vi "CheckSettings.vi"(0 "ChromaAcLoad in":refnum<class "ChromaAcLoad.lvclass">, 1 "RangeCheck":T1, 2 "Phase":i32, 3 "error in (no error)":errorcluster) -> (7 "ChromaAcLoad out":refnum<class "ChromaAcLoad.lvclass">, 10 "error out":errorcluster)   [LabVIEW 2018, in "AcPwrPlugins.lvlib" / "ChromaAcLoad.lvclass"]
doc: "This VI checks the value of the instrument settings and returns an error if the value is outside the instrument range."
uses:
  ChromaAcLoad.lvclass
  C:/Users/ico/Documents/Projects/NistPluggableModules/AcPwr/AcPwrPlugins/AcPwrBaseClass/AcPwrBase.lvclass
  TypeDefs/RangeCheck.ctl
  AcPwrBaseClass/AcPwrBase.lvclass/AcPwrBase.ctl
  AcPwrBaseClass/Accessors/Read BaseConfig.vi
  <vilib>/Utility/error.llb/Error Cluster From Error Code.vi
  <vilib>/ErrorRing/Error Ring.xnode
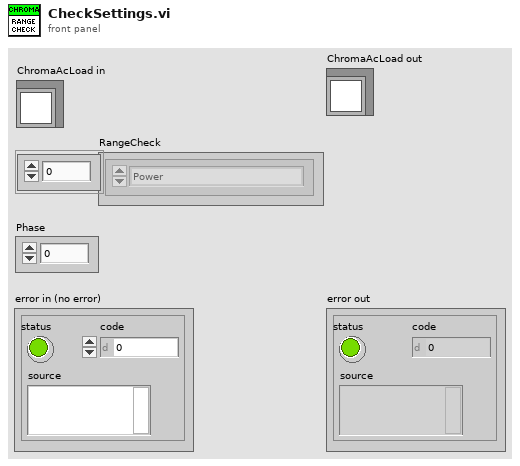
[diagram p1: front panel]
types:
  T1 = typedef "AcPwrPlugins.lvlib/ChromaAcLoad.lvclass/RangeCheck.ctl" = enum16{"Power", "Power Limit", "Current", "Current Peak", "Current Limit", "Voltage", "AC Resistance", "DC Resistance", "Frequency", "Crest Factor", "Power Factor", "RLC Power Factor", "Rise Slew Rate", "Fall Slew Rate", "Capacitance", "Inductance", "Parallel Resistance", "Series Resistance"}[]
  T2 = typedef "AcPwrPlugins.lvlib/AcPwrBase.lvclass/BaseConfig.ctl" = cluster{"Frequency":dbl, "FrequencyRange":dbl[], "Phases":T3[], "Name":string, "Chroma":T4, "NHRDC":T5, "PPS":T6, "PluginConfigVariant":variant}
  T3 = typedef "AcPwrPlugins.lvlib/AcPwrBase.lvclass/Phase.ctl" = cluster{"Name":string, "Enabled":bool, "VoltageLevel":dbl, "Handle":string, "VoltageRange":dbl[], "Connected":bool, "CurrentLimit":dbl, "Waveform":string}
  T4 = typedef "AcPwrPlugins.lvlib/ChromaAcLoad.lvclass/DeviceProperties.ctl" = cluster{"Configuration Mode":enum16{"Constant Voltage (DC)", "Constant Power (DC)", "Constant Power (AC)", "Constant Current (DC)", "Constant Current (AC)", "Constant Resistance (DC)", "Constant Resistance (AC)", "Rectified Mode (DC)", "Inrush (AC)", "RLC CP (AC)", "RLC (AC)"}, "Phases":cluster{"Handle":string, "Name":string, "Phase Select":i32, "Instrument Options":string, "id query (T)":bool, "reset device (T)":bool, "Load Short Circuited":bool, "Line Synchronization":bool, "Load Current (A/Arms)":dbl, "Load Voltage (V/Vrms)":dbl, "Load Power (W)":dbl, "Load Resistance (Ohms)":dbl, "Load Current Peak Limit (A)":dbl, "Load Current Limit (A/Arms)":dbl, "Load Power Limit (W)":dbl, "Synch Frequency (Hz)":dbl, "Priority":enum16{"CF Only", "PF Only", "Both (CF)", "Both (PF)"}, "Crest Factor":dbl, "Power Factor":dbl, "Slew Rate":cluster{"Rise Slew Rate (A/ms)":i32, "Fall Slew Rate (A/ms)":i32}, "LC/RLC Mode":cluster{"Capacitance (uF)":i32, "Inductance (uH)":i32, "Series Resistance (Ohm)":dbl, "Parallel Resistance (Ohm)":dbl}, "Timing":cluster{"TimingOn":enum16{""}, "Hours":u32, "Minutes":u32, "Seconds":dbl, "CutoffVoltage":dbl}, "Connected":bool}[]}
  T5 = typedef "AcPwrPlugins.lvlib/NHRDCPower.lvclass/Device(s)Settings.ctl" = cluster{"Handle":string, "Name":string, "id query (Yes)":bool, "reset device (Yes)":bool, "Connected":bool, "Initial Battery Detect Voltage (0)":sgl, "SafetySettings":cluster{"SetWatchDog":bool, "Voltage (V)":sgl, "Current (A)":sgl, "Power (W)":sgl, "Voltage Delay (s)":sgl, "Current Delay (s)":sgl, "Power Delay (s)":sgl}, "Options String":string, "Aperture Time (s)":sgl, "operating state (Off)":i32, "OutputSettings":cluster{"Voltage (V)":sgl, "Current (A)":sgl, "Resistance (Ohms)":sgl, "Power (W)":sgl, "Enable Voltage":bool, "Enable Current":bool, "Enable Resistance":bool, "Enable Power":bool, "Delay After (s)":sgl, "Wait Value (V, A, W)":sgl, "Enable Wait":bool, "Wait on Value":i32}[], "SlewRate":cluster{"Set Voltage Rate V/S":dbl, "Set Current Rate A/S":dbl, "Set Resistance Rate R/S":dbl, "Set Power Rate W/S":dbl}}[]
  T6 = typedef "AcPwrPlugins.lvlib/PacificPowerSource.lvclass/DeviceSettings.ctl" = cluster{"Handle":string, "Connected":bool, "Clear Device (F)":bool, "btnIdQuery":bool, "btnReset":bool, "Program #":cluster{"Phase B (Degrees)":i32, "Waveform A (1: Sine)":i32, "Voltage Level (Va)":dbl, "Program Number (0)":i32, "Voltage Level (Vb) ":dbl, "Form (3: Three)":u16, "Coupling  (0: Direct)":u16, "Frequency (45Hz)":dbl, "Current Limit (40A)":dbl, "Phase C (Degrees)":i32, "Voltage Level (Vc)":dbl, "Waveform B (1: Sine)":i32, "Waveform C (1: Sine)":i32}[], "Impedance Parameters (off, 0.00)":cluster{"State":bool, "Impedance":dbl}, "Transient Execution (F)":bool, "OutputEnabled":bool, "Source Range":cluster{"Frequency Minimum (45 Hz)":dbl, "Frequency Maximum (1200 Hz)":dbl, "Voltage Maximum (V)":dbl, "Voltage Minimum (V)":dbl, "Range Control (0: Auto)":u16, "Initial Voltage (0V)":u16, "Frequency Range (600Hz)":u16}, "Port Type":enum16{"GPIB", "Serial"}}[]
  T7 = cluster{"Handle":string, "Name":string, "Phase Select":i32, "Instrument Options":string, "id query (T)":bool, "reset device (T)":bool, "Load Short Circuited":bool, "Line Synchronization":bool, "Load Current (A/Arms)":dbl, "Load Voltage (V/Vrms)":dbl, "Load Power (W)":dbl, "Load Resistance (Ohms)":dbl, "Load Current Peak Limit (A)":dbl, "Load Current Limit (A/Arms)":dbl, "Load Power Limit (W)":dbl, "Synch Frequency (Hz)":dbl, "Priority":enum16{"CF Only", "PF Only", "Both (CF)", "Both (PF)"}, "Crest Factor":dbl, "Power Factor":dbl, "Slew Rate":cluster{"Rise Slew Rate (A/ms)":i32, "Fall Slew Rate (A/ms)":i32}, "LC/RLC Mode":cluster{"Capacitance (uF)":i32, "Inductance (uH)":i32, "Series Resistance (Ohm)":dbl, "Parallel Resistance (Ohm)":dbl}, "Timing":cluster{"TimingOn":enum16{""}, "Hours":u32, "Minutes":u32, "Seconds":dbl, "CutoffVoltage":dbl}, "Connected":bool}[]
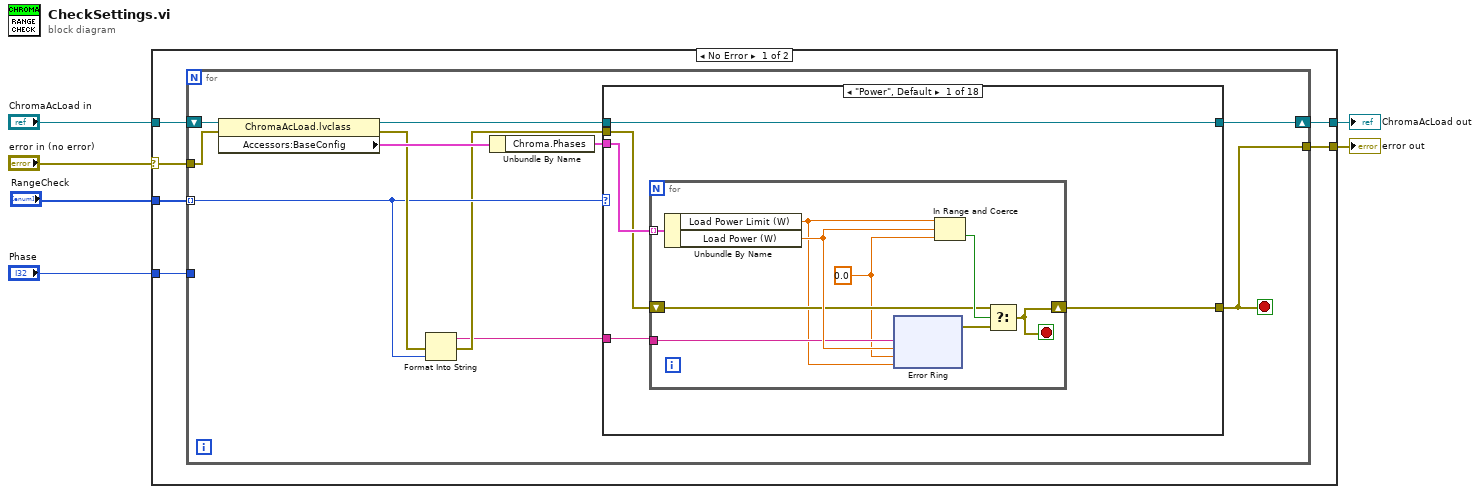
[diagram p0: block diagram]
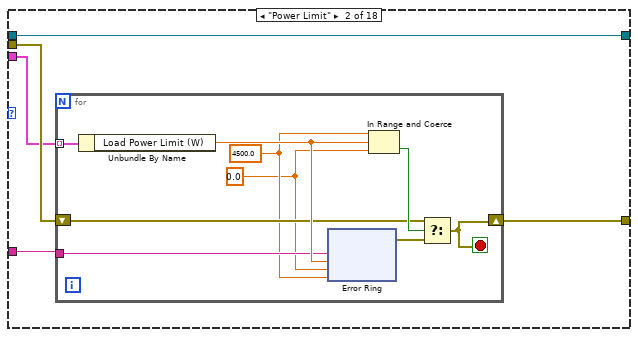
[diagram p2: hidden frame]
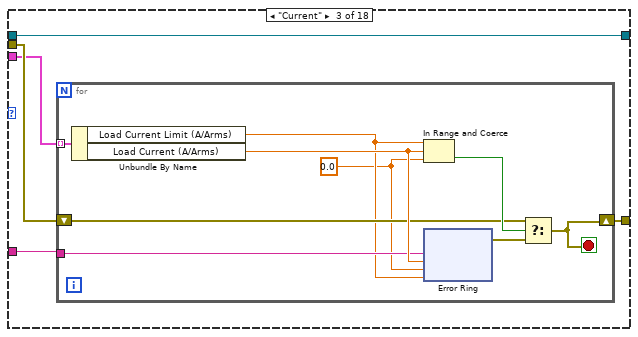
[diagram p3: hidden frame]
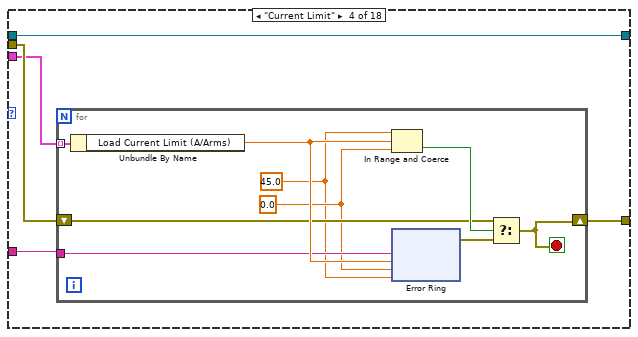
[diagram p4: hidden frame]
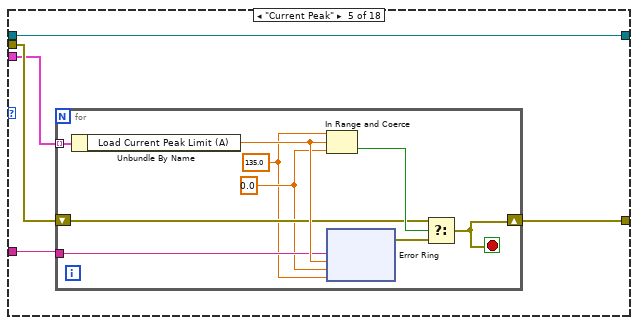
[diagram p5: hidden frame]
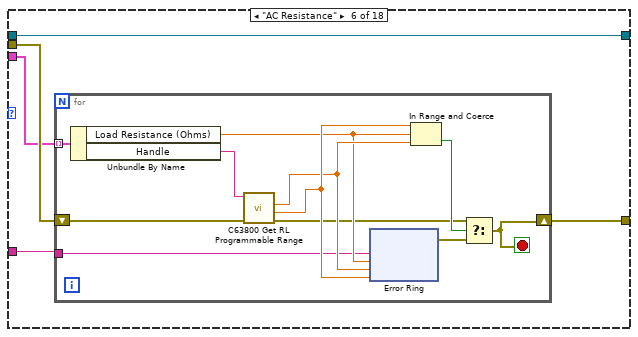
[diagram p6: hidden frame]
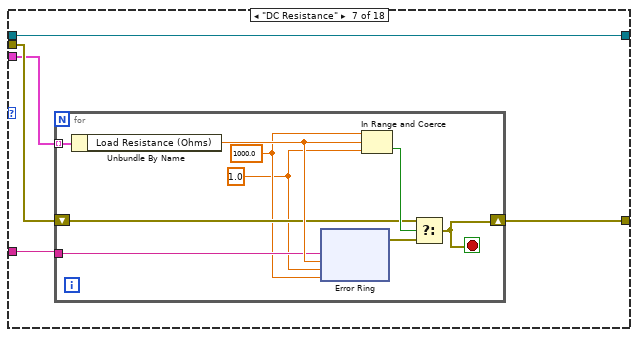
[diagram p7: hidden frame]
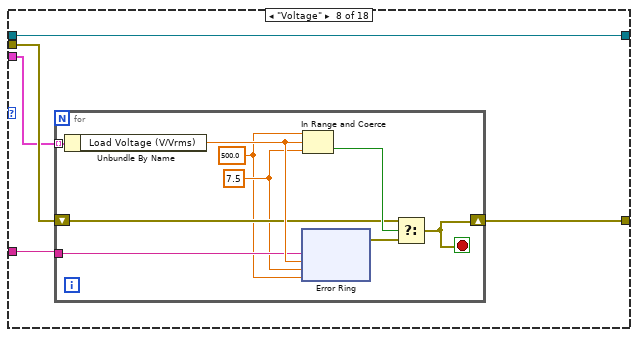
[diagram p8: hidden frame]
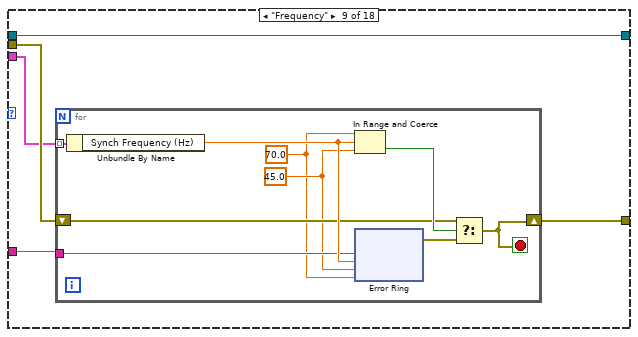
[diagram p9: hidden frame]
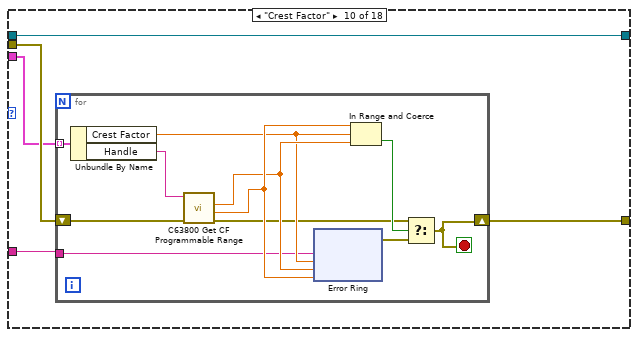
[diagram p10: hidden frame]
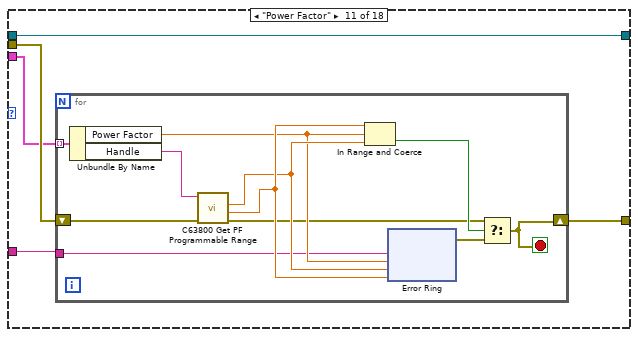
[diagram p11: hidden frame]
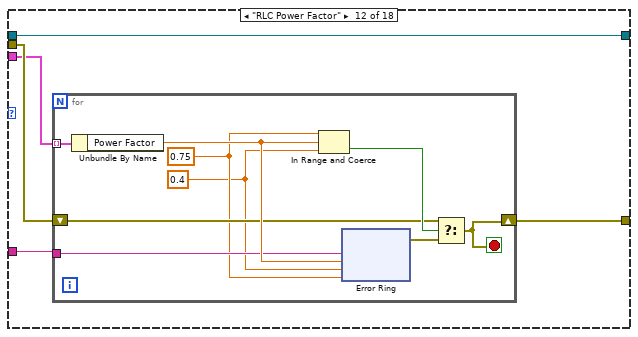
[diagram p12: hidden frame]
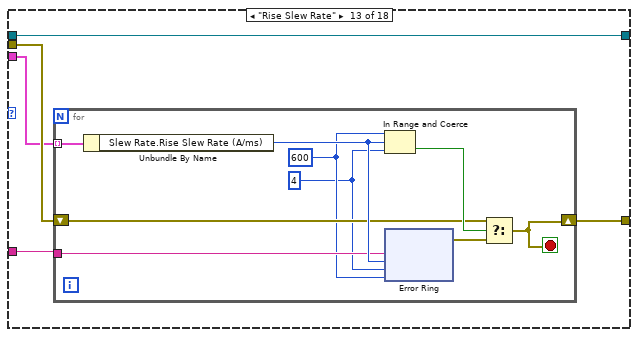
[diagram p13: hidden frame]
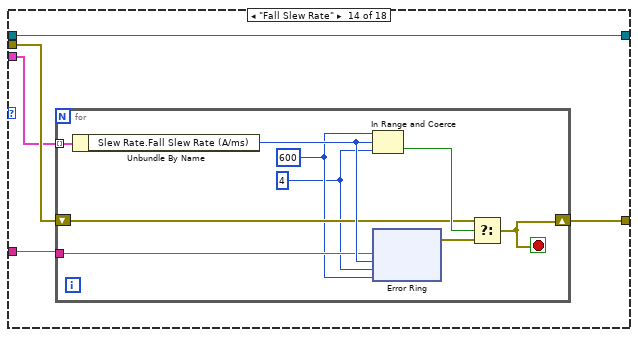
[diagram p14: hidden frame]
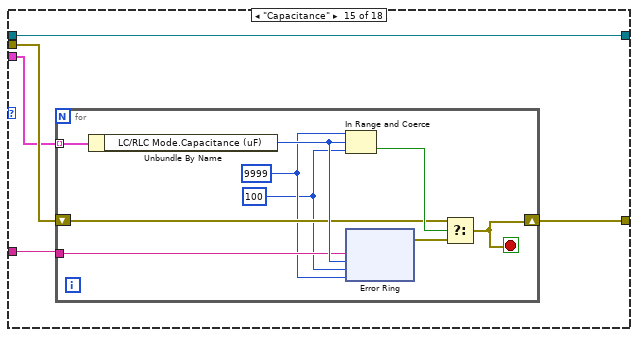
[diagram p15: hidden frame]
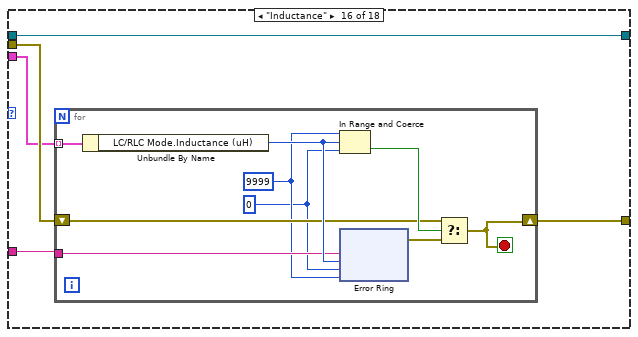
[diagram p16: hidden frame]
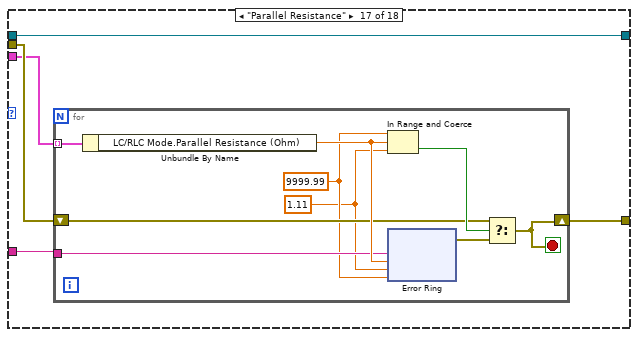
[diagram p17: hidden frame]
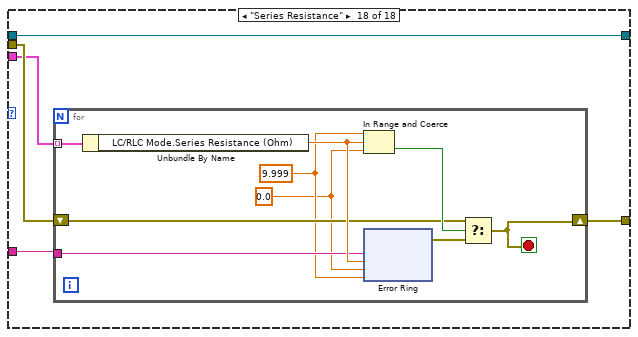
[diagram p18: hidden frame]
diagram:
  n1 = case shown="No Error" "error in (no error)" {
    selector: "error in (no error)" -> [w9 w462]
    tunnel: "ChromaAcLoad in" -> [w12 w463]
    tunnel: "Phase" -> [w11 _]
    tunnel: [w10 w463] -> w4
    tunnel: "RangeCheck" -> [w8 _]
    tunnel: [w7 w462] -> w1
    frame No Error {
      n2 = for {
        tunnel: w11 -> [_]
        shift-right: [w22] -> w10
        shift-left: w12 -> [w20]
        tunnel: w9 -> [w23]
        tunnel: w8 -> [w15] mode=indexing
        tunnel: [w21] -> w7
        stop <- w21 stop-if-true
        n3 = property class="ChromaAcLoad.lvclass"(reference=w20, error in=w23) -> (reference out=w19:refnum<class "ChromaAcLoad.lvclass">, error out=w16:errorcluster, "Accessors:BaseConfig"=w18:T2)
        n4 = Format Into String(error in=w16, w15) -> (resulting string=w13:string, error out=w14:errorcluster)  [unwired: 2 in]
        n5 = Unbundle By Name(w18) -> ("Chroma.Phases"=w17:T7)
        n6 = case shown="\"Power\", Default" w15 {
          tunnel: w19 -> [w28 w52 w76 w100 w124 w148 w174 w198 w222 w246 w272 w298 w322 w346 w370 w394 w418 w442]
          tunnel: w14 -> [w24 w51 w75 w99 w123 w147 w173 w197 w221 w245 w271 w297 w321 w345 w369 w393 w417 w441]
          tunnel: [w28 w52 w76 w100 w124 w148 w174 w198 w222 w246 w272 w298 w322 w346 w370 w394 w418 w442] -> w22
          tunnel: [w27 w50 w74 w98 w122 w146 w172 w196 w220 w244 w270 w296 w320 w344 w368 w392 w416 w440] -> w21
          tunnel: w17 -> [w26 w49 w73 w96 w121 w145 w170 w194 w218 w242 w268 w294 w319 w343 w366 w391 w414 w438]
          tunnel: w13 -> [w25 w48 w72 w97 w120 w144 w171 w195 w219 w243 w269 w295 w318 w342 w367 w390 w415 w439]
          frame "Power", Default {
            n7 = for {
              shift-right: [w34] -> w27
              shift-left: w24 -> [w32]
              tunnel: w26 -> [w36] mode=indexing
              tunnel: w25 -> [w31]
              stop <- w34 stop-if-true
              w29 = 0.0 ("Load Power Limit (W)")
              n8 = Unbundle By Name(w36) -> ("Load Power Limit (W)"=w30:dbl, "Load Power (W)"=w33:dbl)
              n9 = xnode "Error Ring"("parameter 0"=w31, "parameter 1"=w33, "parameter 2"=w29, "parameter 3"=w30) -> ("error out"=w37:errorcluster)
              n10 = In Range and Coerce(upper limit=w30, x=w33, lower limit=w29) -> (In Range?=w35:bool)  [unwired: 1 out]
              n11 = Select(t=w32, s=w35, f=w37) -> (s? t:f=w34:errorcluster)
            }
          }
          frame "Power Limit" {
            n12 = for {
              shift-right: [w58] -> w50
              shift-left: w51 -> [w56]
              tunnel: w49 -> [w60] mode=indexing
              tunnel: w48 -> [w55]
              stop <- w58 stop-if-true
              w54 = 4500.0
              w53 = 0.0
              n13 = Unbundle By Name(w60) -> ("Load Power Limit (W)"=w57:dbl)
              n14 = xnode "Error Ring"("parameter 0"=w55, "parameter 1"=w57, "parameter 2"=w53, "parameter 3"=w54) -> ("error out"=w61:errorcluster)
              n15 = In Range and Coerce(upper limit=w54, x=w57, lower limit=w53) -> (In Range?=w59:bool)  [unwired: 1 out]
              n16 = Select(t=w56, s=w59, f=w61) -> (s? t:f=w58:errorcluster)
            }
          }
          frame "Current" {
            n17 = for {
              shift-right: [w82] -> w74
              shift-left: w75 -> [w80]
              tunnel: w73 -> [w84] mode=indexing
              tunnel: w72 -> [w79]
              stop <- w82 stop-if-true
              w77 = 0.0 ("Load Current (A/Arms)")
              n18 = Unbundle By Name(w84) -> ("Load Current Limit (A/Arms)"=w78:dbl, "Load Current (A/Arms)"=w81:dbl)
              n19 = In Range and Coerce(upper limit=w78, x=w81, lower limit=w77) -> (In Range?=w83:bool)  [unwired: 1 out]
              n20 = xnode "Error Ring"("parameter 0"=w79, "parameter 1"=w81, "parameter 2"=w77, "parameter 3"=w78) -> ("error out"=w85:errorcluster)
              n21 = Select(t=w80, s=w83, f=w85) -> (s? t:f=w82:errorcluster)
            }
          }
          frame "Current Limit" {
            n22 = for {
              shift-right: [w106] -> w98
              shift-left: w99 -> [w104]
              tunnel: w96 -> [w108] mode=indexing
              tunnel: w97 -> [w103]
              stop <- w106 stop-if-true
              w101 = 45.0
              w102 = 0.0
              n23 = Unbundle By Name(w108) -> ("Load Current Limit (A/Arms)"=w105:dbl)
              n24 = In Range and Coerce(upper limit=w101, x=w105, lower limit=w102) -> (In Range?=w107:bool)  [unwired: 1 out]
              n25 = xnode "Error Ring"("parameter 0"=w103, "parameter 1"=w105, "parameter 2"=w102, "parameter 3"=w101) -> ("error out"=w109:errorcluster)
              n26 = Select(t=w104, s=w107, f=w109) -> (s? t:f=w106:errorcluster)
            }
          }
          frame "Current Peak" {
            n27 = for {
              shift-right: [w130] -> w122
              shift-left: w123 -> [w128]
              tunnel: w121 -> [w132] mode=indexing
              tunnel: w120 -> [w127]
              stop <- w130 stop-if-true
              w125 = 135.0
              w126 = 0.0
              n28 = Unbundle By Name(w132) -> ("Load Current Peak Limit (A)"=w129:dbl)
              n29 = In Range and Coerce(upper limit=w125, x=w129, lower limit=w126) -> (In Range?=w131:bool)  [unwired: 1 out]
              n30 = xnode "Error Ring"("parameter 0"=w127, "parameter 1"=w129, "parameter 2"=w126, "parameter 3"=w125) -> ("error out"=w133:errorcluster)
              n31 = Select(t=w128, s=w131, f=w133) -> (s? t:f=w130:errorcluster)
            }
          }
          frame "AC Resistance" {
            n32 = for {
              shift-right: [w154] -> w146
              shift-left: w147 -> [w152]
              tunnel: w145 -> [w158] mode=indexing
              tunnel: w144 -> [w149]
              stop <- w154 stop-if-true
              n33 = Unbundle By Name(w158) -> ("Load Resistance (Ohms)"=w153:dbl, "Handle"=w150:string)
              n34 = call <instrlib>:"C63800 Get RL Programmable Range.vi"("error in (no error)"=w152, "Instrument Handle"=w150) -> ("error out"=w151:errorcluster, "Maximum"=w157:dbl, "Minimum"=w156:dbl)  [unwired: 6 in, 1 out]
              n35 = xnode "Error Ring"("parameter 0"=w149, "parameter 1"=w153, "parameter 2"=w156, "parameter 3"=w157) -> ("error out"=w159:errorcluster)
              n36 = In Range and Coerce(upper limit=w157, x=w153, lower limit=w156) -> (In Range?=w155:bool)  [unwired: 1 out]
              n37 = Select(t=w151, s=w155, f=w159) -> (s? t:f=w154:errorcluster)
            }
          }
          frame "DC Resistance" {
            n38 = for {
              shift-right: [w180] -> w172
              shift-left: w173 -> [w178]
              tunnel: w170 -> [w182] mode=indexing
              tunnel: w171 -> [w177]
              stop <- w180 stop-if-true
              w176 = 1000.0
              w175 = 1.0
              n39 = Unbundle By Name(w182) -> ("Load Resistance (Ohms)"=w179:dbl)
              n40 = xnode "Error Ring"("parameter 0"=w177, "parameter 1"=w179, "parameter 2"=w175, "parameter 3"=w176) -> ("error out"=w183:errorcluster)
              n41 = In Range and Coerce(upper limit=w176, x=w179, lower limit=w175) -> (In Range?=w181:bool)  [unwired: 1 out]
              n42 = Select(t=w178, s=w181, f=w183) -> (s? t:f=w180:errorcluster)
            }
          }
          frame "Voltage" {
            n43 = for {
              shift-right: [w204] -> w196
              shift-left: w197 -> [w202]
              tunnel: w194 -> [w206] mode=indexing
              tunnel: w195 -> [w201]
              stop <- w204 stop-if-true
              w199 = 500.0
              w200 = 7.5
              n44 = Unbundle By Name(w206) -> ("Load Voltage (V/Vrms)"=w203:dbl)
              n45 = xnode "Error Ring"("parameter 0"=w201, "parameter 1"=w203, "parameter 2"=w200, "parameter 3"=w199) -> ("error out"=w207:errorcluster)
              n46 = In Range and Coerce(upper limit=w199, x=w203, lower limit=w200) -> (In Range?=w205:bool)  [unwired: 1 out]
              n47 = Select(t=w202, s=w205, f=w207) -> (s? t:f=w204:errorcluster)
            }
          }
          frame "Frequency" {
            n48 = for {
              shift-right: [w228] -> w220
              shift-left: w221 -> [w226]
              tunnel: w218 -> [w230] mode=indexing
              tunnel: w219 -> [w225]
              stop <- w228 stop-if-true
              w223 = 70.0 ("Minimum")
              w224 = 45.0 ("Minimum")
              n49 = Unbundle By Name(w230) -> ("Synch Frequency (Hz)"=w227:dbl)
              n50 = In Range and Coerce(upper limit=w223, x=w227, lower limit=w224) -> (In Range?=w229:bool)  [unwired: 1 out]
              n51 = xnode "Error Ring"("parameter 0"=w225, "parameter 1"=w227, "parameter 2"=w224, "parameter 3"=w223) -> ("error out"=w231:errorcluster)
              n52 = Select(t=w226, s=w229, f=w231) -> (s? t:f=w228:errorcluster)
            }
          }
          frame "Crest Factor" {
            n53 = for {
              shift-right: [w252] -> w244
              shift-left: w245 -> [w250]
              tunnel: w242 -> [w256] mode=indexing
              tunnel: w243 -> [w247]
              stop <- w252 stop-if-true
              n54 = Unbundle By Name(w256) -> ("Crest Factor"=w251:dbl, "Handle"=w248:string)
              n55 = call <instrlib>:"C63800 Get CF Programmable Range.vi"("error in (no error)"=w250, "Instrument Handle"=w248) -> ("error out"=w249:errorcluster, "Maximum"=w255:dbl, "Minimum"=w254:dbl)  [unwired: 6 in, 1 out]
              n56 = xnode "Error Ring"("parameter 0"=w247, "parameter 1"=w251, "parameter 2"=w254, "parameter 3"=w255) -> ("error out"=w257:errorcluster)
              n57 = In Range and Coerce(upper limit=w255, x=w251, lower limit=w254) -> (In Range?=w253:bool)  [unwired: 1 out]
              n58 = Select(t=w249, s=w253, f=w257) -> (s? t:f=w252:errorcluster)
            }
          }
          frame "Power Factor" {
            n59 = for {
              shift-right: [w278] -> w270
              shift-left: w271 -> [w276]
              tunnel: w268 -> [w282] mode=indexing
              tunnel: w269 -> [w273]
              stop <- w278 stop-if-true
              n60 = Unbundle By Name(w282) -> ("Power Factor"=w277:dbl, "Handle"=w274:string)
              n61 = call <instrlib>:"C63800 Get PF Programmable Range.vi"("error in (no error)"=w276, "Instrument Handle"=w274) -> ("error out"=w275:errorcluster, "Maximum"=w281:dbl, "Minimum"=w280:dbl)  [unwired: 6 in, 1 out]
              n62 = In Range and Coerce(upper limit=w281, x=w277, lower limit=w280) -> (In Range?=w279:bool)  [unwired: 1 out]
              n63 = xnode "Error Ring"("parameter 0"=w273, "parameter 1"=w277, "parameter 2"=w280, "parameter 3"=w281) -> ("error out"=w283:errorcluster)
              n64 = Select(t=w275, s=w279, f=w283) -> (s? t:f=w278:errorcluster)
            }
          }
          frame "RLC Power Factor" {
            n65 = for {
              shift-right: [w304] -> w296
              shift-left: w297 -> [w302]
              tunnel: w294 -> [w306] mode=indexing
              tunnel: w295 -> [w301]
              stop <- w304 stop-if-true
              w300 = 0.75
              w299 = 0.4
              n66 = Unbundle By Name(w306) -> ("Power Factor"=w303:dbl)
              n67 = In Range and Coerce(upper limit=w300, x=w303, lower limit=w299) -> (In Range?=w305:bool)  [unwired: 1 out]
              n68 = xnode "Error Ring"("parameter 0"=w301, "parameter 1"=w303, "parameter 2"=w299, "parameter 3"=w300) -> ("error out"=w307:errorcluster)
              n69 = Select(t=w302, s=w305, f=w307) -> (s? t:f=w304:errorcluster)
            }
          }
          frame "Rise Slew Rate" {
            n70 = for {
              shift-right: [w328] -> w320
              shift-left: w321 -> [w326]
              tunnel: w319 -> [w330] mode=indexing
              tunnel: w318 -> [w325]
              stop <- w328 stop-if-true
              w324 = 600
              w323 = 4
              n71 = Unbundle By Name(w330) -> ("Slew Rate.Rise Slew Rate (A/ms)"=w327:i32)
              n72 = In Range and Coerce(upper limit=w324, x=w327, lower limit=w323) -> (In Range?=w329:bool)  [unwired: 1 out]
              n73 = xnode "Error Ring"("parameter 0"=w325, "parameter 1"=w327, "parameter 2"=w323, "parameter 3"=w324) -> ("error out"=w331:errorcluster)
              n74 = Select(t=w326, s=w329, f=w331) -> (s? t:f=w328:errorcluster)
            }
          }
          frame "Fall Slew Rate" {
            n75 = for {
              shift-right: [w352] -> w344
              shift-left: w345 -> [w350]
              tunnel: w343 -> [w354] mode=indexing
              tunnel: w342 -> [w349]
              stop <- w352 stop-if-true
              w348 = 600
              w347 = 4
              n76 = Unbundle By Name(w354) -> ("Slew Rate.Fall Slew Rate (A/ms)"=w351:i32)
              n77 = In Range and Coerce(upper limit=w348, x=w351, lower limit=w347) -> (In Range?=w353:bool)  [unwired: 1 out]
              n78 = xnode "Error Ring"("parameter 0"=w349, "parameter 1"=w351, "parameter 2"=w347, "parameter 3"=w348) -> ("error out"=w355:errorcluster)
              n79 = Select(t=w350, s=w353, f=w355) -> (s? t:f=w352:errorcluster)
            }
          }
          frame "Capacitance" {
            n80 = for {
              shift-right: [w376] -> w368
              shift-left: w369 -> [w374]
              tunnel: w366 -> [w378] mode=indexing
              tunnel: w367 -> [w373]
              stop <- w376 stop-if-true
              w372 = 9999
              w371 = 100
              n81 = Unbundle By Name(w378) -> ("LC/RLC Mode.Capacitance (uF)"=w375:i32)
              n82 = In Range and Coerce(upper limit=w372, x=w375, lower limit=w371) -> (In Range?=w377:bool)  [unwired: 1 out]
              n83 = xnode "Error Ring"("parameter 0"=w373, "parameter 1"=w375, "parameter 2"=w371, "parameter 3"=w372) -> ("error out"=w379:errorcluster)
              n84 = Select(t=w374, s=w377, f=w379) -> (s? t:f=w376:errorcluster)
            }
          }
          frame "Inductance" {
            n85 = for {
              shift-right: [w400] -> w392
              shift-left: w393 -> [w398]
              tunnel: w391 -> [w402] mode=indexing
              tunnel: w390 -> [w397]
              stop <- w400 stop-if-true
              w396 = 9999
              w395 = 0
              n86 = Unbundle By Name(w402) -> ("LC/RLC Mode.Inductance (uH)"=w399:i32)
              n87 = In Range and Coerce(upper limit=w396, x=w399, lower limit=w395) -> (In Range?=w401:bool)  [unwired: 1 out]
              n88 = xnode "Error Ring"("parameter 0"=w397, "parameter 1"=w399, "parameter 2"=w395, "parameter 3"=w396) -> ("error out"=w403:errorcluster)
              n89 = Select(t=w398, s=w401, f=w403) -> (s? t:f=w400:errorcluster)
            }
          }
          frame "Parallel Resistance" {
            n90 = for {
              shift-right: [w424] -> w416
              shift-left: w417 -> [w422]
              tunnel: w414 -> [w426] mode=indexing
              tunnel: w415 -> [w421]
              stop <- w424 stop-if-true
              w420 = 9999.99
              w419 = 1.11
              n91 = Unbundle By Name(w426) -> ("LC/RLC Mode.Parallel Resistance (Ohm)"=w423:dbl)
              n92 = In Range and Coerce(upper limit=w420, x=w423, lower limit=w419) -> (In Range?=w425:bool)  [unwired: 1 out]
              n93 = xnode "Error Ring"("parameter 0"=w421, "parameter 1"=w423, "parameter 2"=w419, "parameter 3"=w420) -> ("error out"=w427:errorcluster)
              n94 = Select(t=w422, s=w425, f=w427) -> (s? t:f=w424:errorcluster)
            }
          }
          frame "Series Resistance" {
            n95 = for {
              shift-right: [w448] -> w440
              shift-left: w441 -> [w446]
              tunnel: w438 -> [w450] mode=indexing
              tunnel: w439 -> [w445]
              stop <- w448 stop-if-true
              w444 = 9.999
              w443 = 0.0
              n96 = Unbundle By Name(w450) -> ("LC/RLC Mode.Series Resistance (Ohm)"=w447:dbl)
              n97 = In Range and Coerce(upper limit=w444, x=w447, lower limit=w443) -> (In Range?=w449:bool)  [unwired: 1 out]
              n98 = xnode "Error Ring"("parameter 0"=w445, "parameter 1"=w447, "parameter 2"=w443, "parameter 3"=w444) -> ("error out"=w451:errorcluster)
              n99 = Select(t=w446, s=w449, f=w451) -> (s? t:f=w448:errorcluster)
            }
          }
        }
      }
    }
    frame Error {
    }
  }
  "error out" <- w1
  "ChromaAcLoad out" <- w4
